vi "foor.vi"() -> ()   [LabVIEW 2020]
uses:
  fooristaatus.ctl
panel:
  out "roheline":bool
  out "kollane":bool
  out "punane":bool
  in  "stop":bool
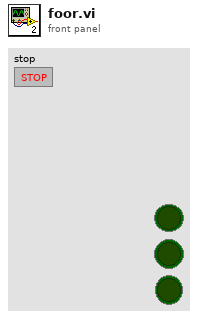
[diagram p1: front panel]
types:
  T1 = typedef "fooristaatus.ctl" = enum16{"Punane", "Kollane", "Roheline"}
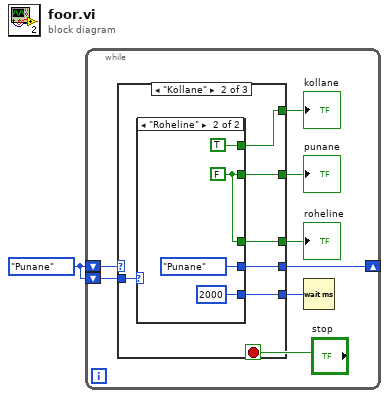
[diagram p0: block diagram]
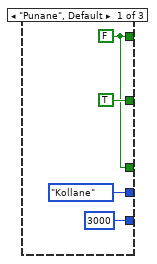
[diagram p2: hidden frame]
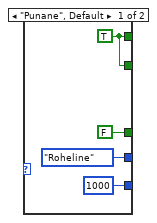
[diagram p3: hidden frame]
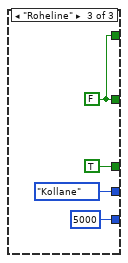
[diagram p4: hidden frame]
diagram:
  w1 = fooristaatus."Punane"
  n1 = while {
    shift-right: [w9] -> _
    shift-left: w1 -> [w3]
    shift-left: w1 -> [w5]
    stop <- "stop" stop-if-true
    n2 = case shown="\"Kollane\"" w3 {
      tunnel: [fooristaatus."Kollane" w19 fooristaatus."Kollane"] -> w9
      tunnel: [TRUE w14 w29] -> w8
      tunnel: [w11 w16 TRUE] -> w7
      tunnel: [w11 w15 w29] -> w6
      tunnel: w5 -> [_ w17 _]
      tunnel: [u32 3000 ("milliseconds to wait") w18 u32 5000 ("milliseconds to wait")] -> w4
      frame "Punane", Default {
        w11 = FALSE
      }
      frame "Kollane" {
        n3 = case shown="\"Roheline\"" w17 {
          tunnel: [fooristaatus."Roheline" fooristaatus."Punane"] -> w19
          tunnel: [w22 TRUE] -> w15
          tunnel: [w22 w26] -> w14
          tunnel: [FALSE w26] -> w16
          tunnel: [u32 1000 ("milliseconds to wait") u32 2000 ("milliseconds to wait")] -> w18
          frame "Punane", Default {
            w22 = TRUE
          }
          frame "Roheline" {
            w26 = FALSE
          }
        }
      }
      frame "Roheline" {
        w29 = FALSE
      }
    }
    "punane" <- w8
    "roheline" <- w7
    "kollane" <- w6
    n4 = Wait (ms)(milliseconds to wait=w4) -> ()  [unwired: 1 out]
  }
